vi "Register Field Value Change Events.vi"(8 "error in (no error)":errorcluster, 10 "Field Event Refnum In":refnum<event-registration>, 11 "Panel Form Controller in":refnum<class "Panel Form Controller.lvclass">) -> (0 "error out":errorcluster, 2 "Field Event Refnum Out":refnum<event-registration>, 3 "Panel Form Controller out":refnum<class "Panel Form Controller.lvclass">)   [LabVIEW 2020, in "Panel Form Controller.lvlib" / "Panel Form Controller.lvclass"]
uses:
  Panel Form Controller.lvclass
  Panel Form Controller.lvclass/Panel Form Controller.ctl
  Database OOP/Table Libraries/Basic Form/Basic Form.lvclass
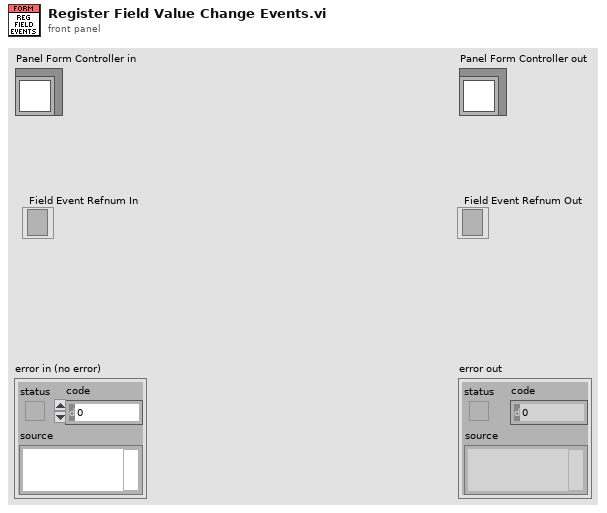
[diagram p1: front panel]
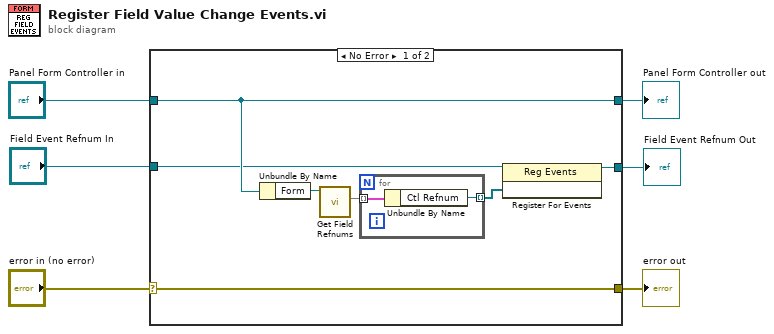
[diagram p0: block diagram]
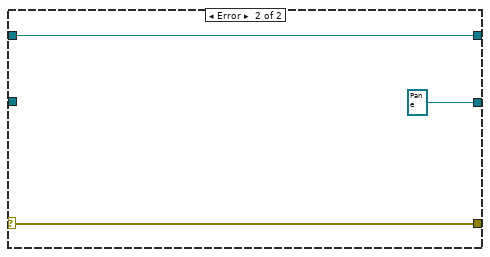
[diagram p2: hidden frame]
diagram:
  n1 = case shown="No Error" "error in (no error)" {
    selector: "error in (no error)" -> [w13 w18]
    tunnel: [w13 w18] -> w5
    tunnel: [w12 w17] -> w3
    tunnel: "Panel Form Controller in" -> [w12 w17]
    tunnel: [w11 refnum<event-registration> refnum ("field value change")] -> w2
    tunnel: "Field Event Refnum In" -> [w10 _]
    frame No Error {
      n2 = Unbundle By Name(w12) -> ("Form"=w9:refnum<class "Basic Form.lvclass">)
      n3 = call "Get Field Refnums.vi"("Basic Form in"=w9) -> ("Field Refnums"=w8:map{string, refnum<vi>})  [unwired: 8 in, 2 out]
      n4 = for {
        tunnel: w8 -> [w15] mode=indexing
        tunnel: [w14] -> w7 mode=indexing
        n5 = Unbundle By Name(w15) -> ("Ctl Refnum"=w14:refnum<vi>)
      }
      n6 = register-events(reference=w10, w7) -> (reference out=w11:refnum<event-registration>)  [unwired: 1 in, 1 out]
    }
    frame Error {
    }
  }
  "error out" <- w5
  "Panel Form Controller out" <- w3
  "Field Event Refnum Out" <- w2
